vi "update_dict_HIS_selected_images.vi"(6 "Select":bool, 8 "error in (no error)":errorcluster, 9 "All":bool, 10 "type":string, 11 "dict of HIS IN":variant) -> (0 "error out":errorcluster, 3 "dict of HIS OUT":variant)   [LabVIEW 2015]
uses:
  cluster_template.ctl
  Classes/DATA/HIS/HIS.lvclass
  Classes/DATA/DATA.lvclass/DATA.ctl
  Classes/DATA/HIS/HIS.lvclass/HIS.ctl
  <userlib>/_OpenG.lib/array/array.llb/Sort 1D Array (I32)__ogtk.vi
  <userlib>/_OpenG.lib/array/array.llb/Filter 1D Array (I32)__ogtk.vi
  Classes/DATA/DATA.lvclass
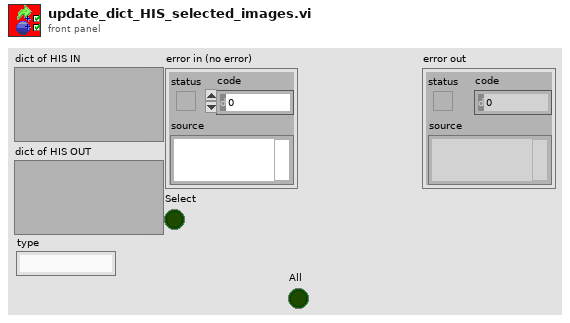
[diagram p1: front panel]
types:
  T1 = typedef "cluster_template.ctl" = cluster{"HIS.lvclass":refnum<class "HIS.lvclass">, "selector":refnum<vi>, "HIS graph":refnum<vi>, "DAT graph":refnum<vi>, "path":refnum<vi>, "path MAIN":refnum<vi>, "#":refnum<vi>, "unsel Graph":refnum<vi>, "DATgraph":refnum<vi>}
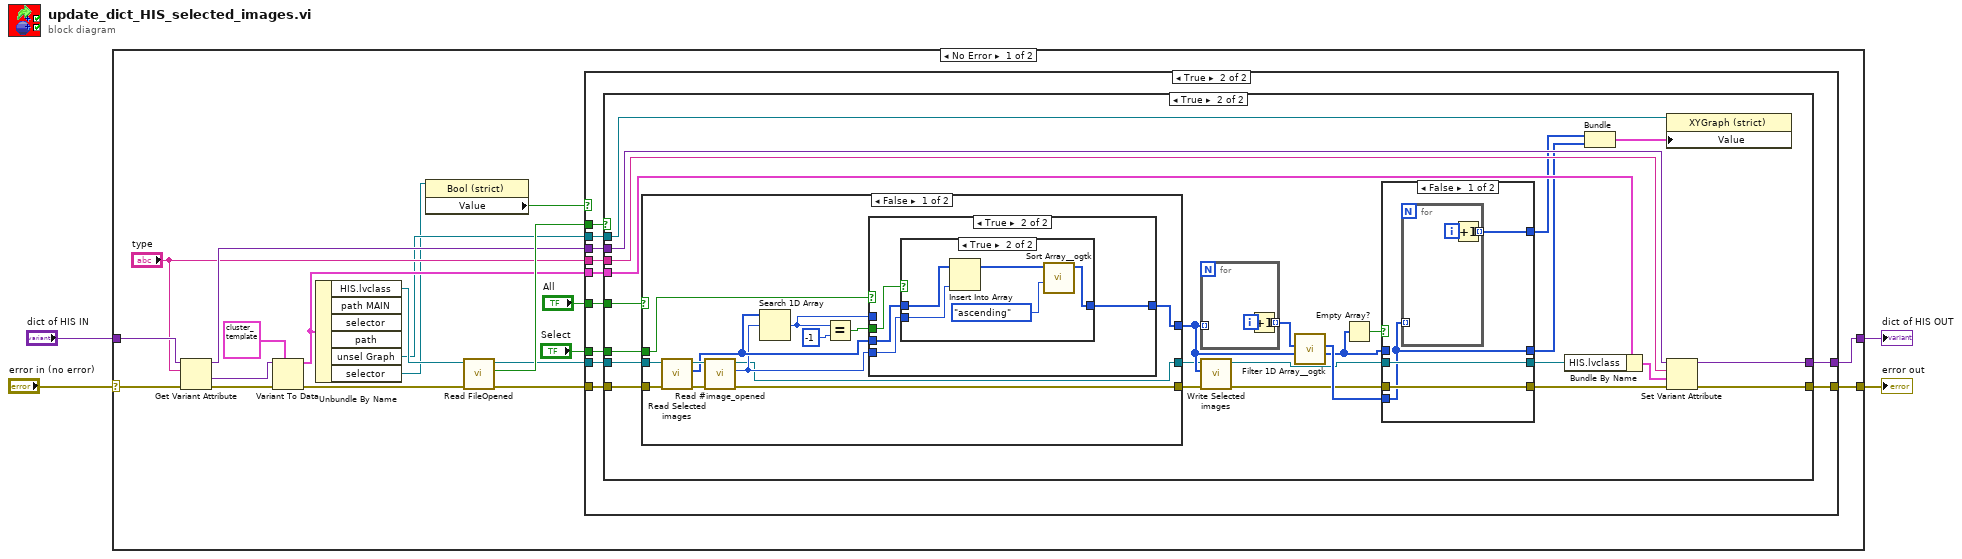
[diagram p0: block diagram]
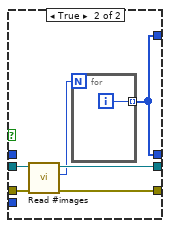
[diagram p4: hidden frame]
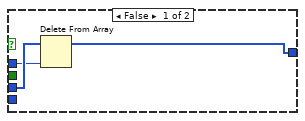
[diagram p5: hidden frame]
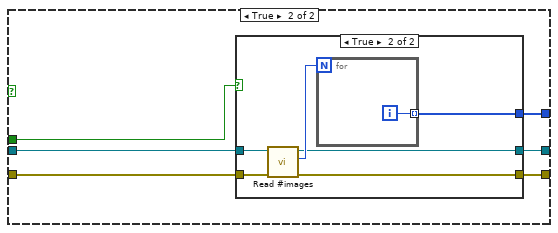
[diagram p7: hidden frame]
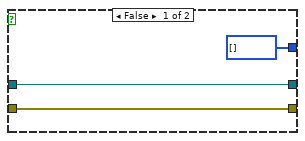
[diagram p8: hidden frame]
diagram:
  n1 = case shown="No Error" "error in (no error)" {
    selector: "error in (no error)" -> [w23 w123]
    tunnel: "dict of HIS IN" -> [w24 w122]
    tunnel: [w13 w122] -> w3
    tunnel: [w11 w123] -> w2
    frame No Error {
      n2 = Get Variant Attribute(Variant=w24, name="type", error in=w23) -> (duplicate Variant=w12:variant, value=w22:variant, error out=w21:errorcluster)  [unwired: 1 in, 1 out]
      n3 = Variant To Data(error in=w21, type=T1 {"HIS.lvclass"=refnum, "selector"=refnum, "HIS graph"=refnum, "DAT graph"=refnum, "path"=refnum, "path MAIN"=refnum, "#"=refnum, "unsel Graph"=refnum, "DATgraph"=refnum} ("output cluster"), Variant=w22) -> (data=w14:T1, error out=w18:errorcluster)
      n4 = Unbundle By Name(w14) -> ("HIS.lvclass"=w19:refnum<class "HIS.lvclass">, "unsel Graph"=w7:refnum<vi>, "selector"=w6:refnum<vi>)  [unwired: 3 out]
      n5 = property class="Bool (strict)"(reference=w6) -> ("Value"=w5:bool)  [unwired: 1 in, 2 out]
      n6 = call "Read FileOpened.vi"("error in (no error)"=w18, "DATA in"=w19) -> ("error out"=w15:errorcluster, "FileOpened"=w17:bool, "DATA out"=w16:refnum<class "HIS.lvclass">)  [unwired: 7 in]
      n7 = case shown="True" w5 {
        tunnel: w17 -> [_ w37]
        tunnel: w16 -> [_ w36]
        tunnel: w15 -> [w25 w35]
        tunnel: w14 -> [_ w34]
        tunnel: [w26 w33] -> w13
        tunnel: w12 -> [w26 w32]
        tunnel: [w25 w31] -> w11
        tunnel: "type" -> [_ w30]
        tunnel: "All" -> [_ w29]
        tunnel: "Select" -> [_ w28]
        tunnel: w7 -> [_ w27]
        frame False {
        }
        frame True {
          n8 = case shown="True" w37 {
            tunnel: w36 -> [_ w57]
            tunnel: w35 -> [w39 w58]
            tunnel: [w39 w62] -> w31
            tunnel: w34 -> [_ w63]
            tunnel: [w38 w61] -> w33
            tunnel: w32 -> [w38 w60]
            tunnel: w30 -> [_ w59]
            tunnel: w29 -> [_ w56]
            tunnel: w28 -> [_ w55]
            tunnel: w27 -> [_ w53]
            frame False {
            }
            frame True {
              n9 = case shown="False" w56 {
                tunnel: w58 -> [w92 w111]
                tunnel: w57 -> [w91 w110]
                tunnel: w55 -> [w83 w109]
                tunnel: [w84 w108] -> w51
                tunnel: [w81 w106] -> w54
                tunnel: [w80 w107] -> w46
                frame False {
                  n10 = call "Read Selected images.vi"("error in (no error)"=w92, "HIS in"=w91) -> ("error out"=w89:errorcluster, "Selected images"=w86:i32[], "HIS out"=w90:refnum<class "HIS.lvclass">)  [unwired: 7 in]
                  n11 = call "Read #image_opened.vi"("error in (no error)"=w89, "HIS in"=w90) -> ("error out"=w81:errorcluster, "#image_opened"=w85:i32, "HIS out"=w80:refnum<class "HIS.lvclass">)  [unwired: 7 in]
                  n12 = Search 1D Array(1D array=w86, element=w85) -> (index of element=w82:i32)  [unwired: 1 in]
                  n13 = Equal?(x=w82, y=-1) -> (x = y?=w87:bool)
                  n14 = case shown="True" w83 {
                    tunnel: w87 -> [_ w99]
                    tunnel: w86 -> [w95 w98]
                    tunnel: w85 -> [_ w97]
                    tunnel: [w93 w96] -> w84
                    tunnel: w82 -> [w94 _]
                    frame False {
                      n15 = Delete From Array(array=w95, index=w94) -> (array with subset deleted=w93:i32[])  [unwired: 1 in, 1 out]
                    }
                    frame True {
                      n16 = case shown="True" w99 {
                        tunnel: w98 -> [w100 w105]
                        tunnel: w97 -> [_ w104]
                        tunnel: [w100 w101] -> w96
                        frame False {
                        }
                        frame True {
                          n17 = Insert Into Array(array=w105, new element=w104) -> (w103:i32[])  [unwired: 1 in]
                          n18 = call-poly <userlib>:"Sort Array__ogtk.vi"("Order"=enum16{"ascending", "descending"}."ascending", "Array in"=w103) -> ("Sorted Array out"=w101:i32[])  [unwired: 8 in, 1 out]
                        }
                      }
                    }
                  }
                }
                frame True {
                  n19 = case shown="True" w109 {
                    tunnel: w111 -> [w112 w120]
                    tunnel: w110 -> [w113 w119]
                    tunnel: [i32[] [] w117] -> w108
                    tunnel: [w113 w116] -> w107
                    tunnel: [w112 w115] -> w106
                    frame False {
                    }
                    frame True {
                      n20 = call "Read #images.vi"("error in (no error)"=w120, "HIS in"=w119) -> ("error out"=w115:errorcluster, "#images"=w118:i32, "HIS out"=w116:refnum<class "HIS.lvclass">)  [unwired: 7 in]
                      n21 = for {
                        N: w118 -> [_]
                        tunnel: [w121] -> w117 mode=indexing
                        i -> [w121]
                      }
                    }
                  }
                }
              }
              n22 = for {
                tunnel: w51 -> [_] mode=indexing
                tunnel: [w78] -> w50 mode=indexing
                i -> [w79]
                n23 = Increment(x=w79) -> (x+1=w78:i32)
              }
              n24 = call "Write Selected images.vi"("error in (no error)"=w54, "Selected images"=w51, "HIS in"=w46) -> ("error out"=w43:errorcluster, "HIS out"=w45:refnum<class "HIS.lvclass">)  [unwired: 7 in]
              n25 = call-poly <userlib>:"Filter 1D Array__ogtk.vi"("items to filter"=w51, "array"=w50) -> ("filtered item indices"=w40:i32[], "filtered array"=w48:i32[])  [unwired: 4 in]
              n26 = Empty Array?(array=w40) -> (empty?=w47:bool)
              n27 = case shown="False" w47 {
                tunnel: w48 -> [w65 _]
                tunnel: [w68 w71] -> w49
                tunnel: w45 -> [w67 w76]
                tunnel: [w67 w75] -> w44
                tunnel: w43 -> [w66 w74]
                tunnel: [w66 w73] -> w42
                tunnel: [w65 w71] -> w41
                tunnel: w40 -> [_ _]
                frame False {
                  n28 = for {
                    tunnel: w65 -> [_] mode=indexing
                    tunnel: [w69] -> w68 mode=indexing
                    i -> [w70]
                    n29 = Increment(x=w70) -> (x+1=w69:i32)
                  }
                }
                frame True {
                  n30 = call "Read #images.vi"("error in (no error)"=w74, "HIS in"=w76) -> ("error out"=w73:errorcluster, "#images"=w72:i32, "HIS out"=w75:refnum<class "HIS.lvclass">)  [unwired: 7 in]
                  n31 = for {
                    N: w72 -> [_]
                    tunnel: [w77] -> w71 mode=indexing
                    i -> [w77]
                  }
                }
              }
              n32 = Bundle By Name(cluster=w63, "HIS.lvclass"=w44) -> (w64:T1)
              n33 = Bundle(w49, "filtered array"=w41) -> (w52:cluster{i32[], "filtered array":i32[]})  [unwired: 1 in]
              n34 = property class="XYGraph (strict)"(reference=w53, "Value"=w52) -> ()  [unwired: 1 in, 2 out]
              n35 = Set Variant Attribute(Variant=w60, name=w59, value=w64, error in=w42) -> (Variant out=w61:variant, error out=w62:errorcluster)  [unwired: 1 out]
            }
          }
        }
      }
    }
    frame Error {
    }
  }
  "dict of HIS OUT" <- w3
  "error out" <- w2
